vi "Add Constant or Error VI.vi"() -> ()   [LabVIEW 2020, in "ConstantErrorsMaker.lvlib"]
uses:
  Libraries/ConstantErrorsMaker/ConstantErrorsMaker.lvlib
  Libraries/ConstantErrorsMaker/VI to make Type--enum.ctl
panel:
  in  "Selection":T1
  in  "Cancel":bool
  in  "OK":bool
  in  "Target":u16(ring) items=["Project : To Test PDash.lvproj", "Library : My Singleton Module.lvlib", "Library : My Cloneable Module.lvlib", "Library : Application.lvlib", "Library : ConstantErrorsMaker.lvlib", "Class : SingletonClass.lvclass", "Class : CloneableClass.lvclass", "Class : Project Class.lvclass", "<Select a Module/Library/Project>"]
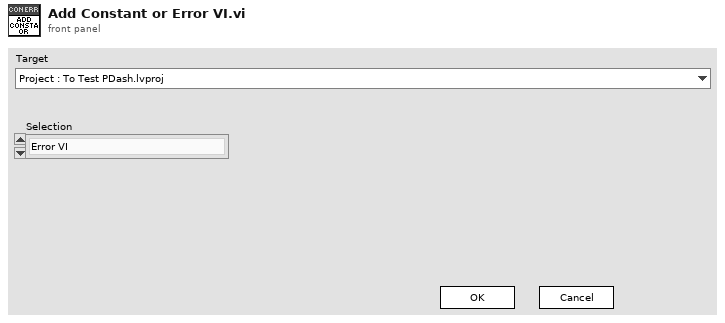
[diagram p1: front panel]
types:
  T1 = typedef "ConstantErrorsMaker.lvlib/VI to make Type--enum.ctl" = enum16{"Error VI", "Constant VI"}
  T2 = typedef "ConstantErrorsMaker.lvlib/Selection Info--cluster.ctl" = cluster{"Name":string, "Library Ref":refnum<vi>, "Application Instance":refnum<vi>, "Selection Owning Folder":path, "Selection Type":T3, "Project Reference":refnum<vi>, "LVClassLibrary Refnum":refnum<vi>}
  T3 = typedef "ConstantErrorsMaker.lvlib/Selection Type--enum.ctl" = enum16{"Project", "Library", "Class"}
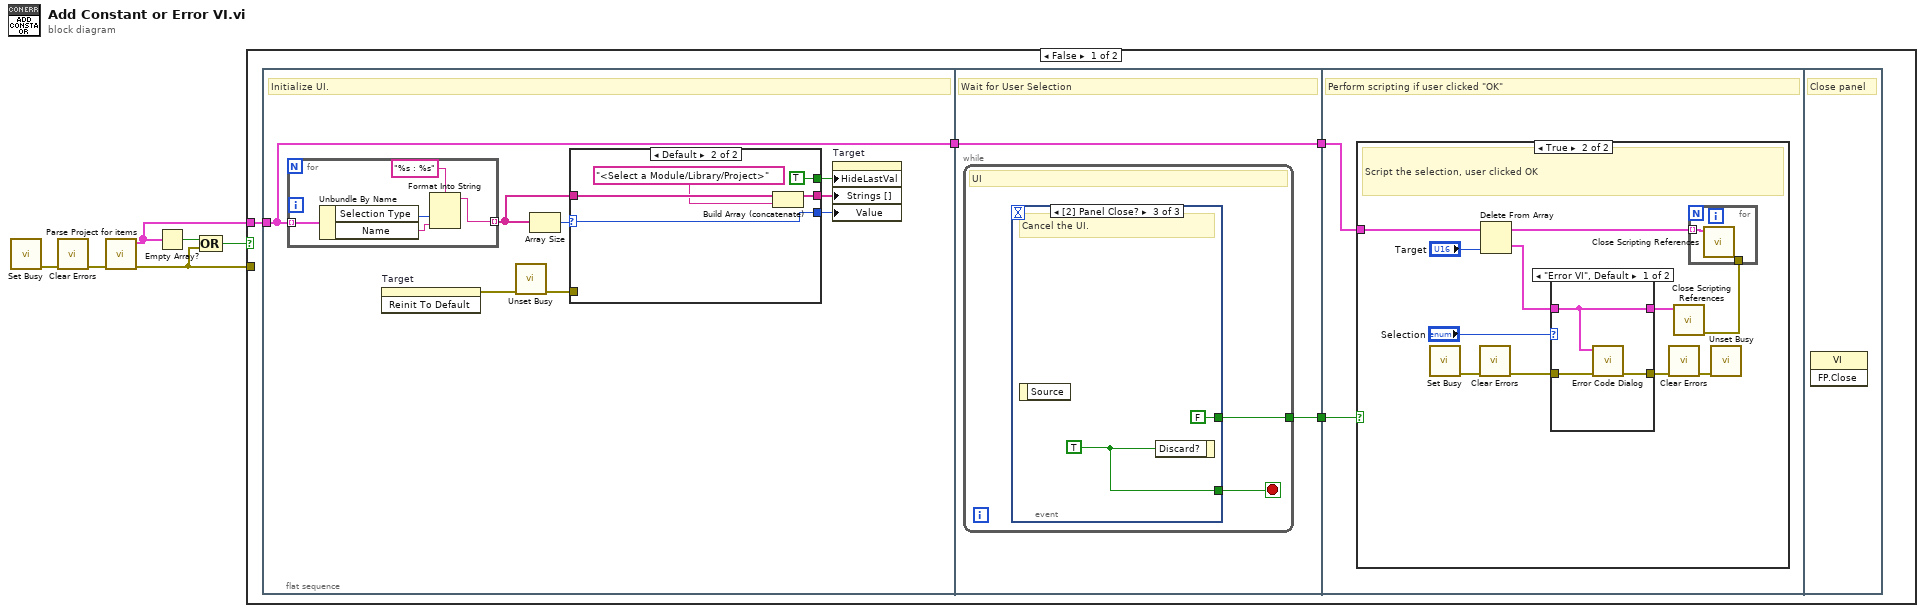
[diagram p0: block diagram]
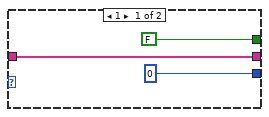
[diagram p2: hidden frame]
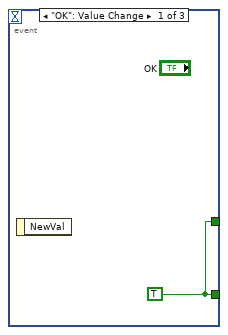
[diagram p3: hidden frame]
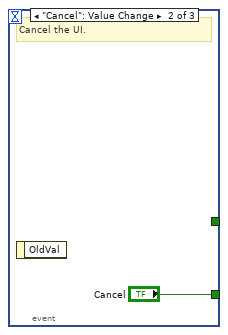
[diagram p4: hidden frame]
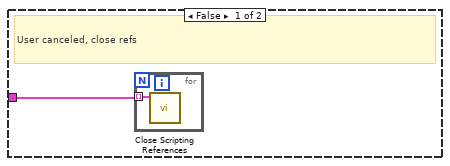
[diagram p5: hidden frame]
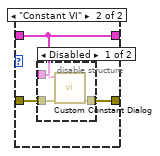
[diagram p6: hidden frame]
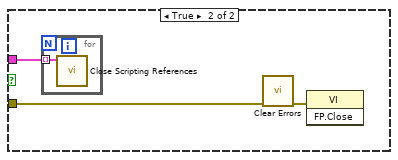
[diagram p8: hidden frame]
diagram:
  n1 = call <vilib>:"Set Busy.vi"() -> ("error out"=w5:errorcluster)  [unwired: 10 in, 1 out]
  n2 = call <vilib>:"Clear Errors.vi"("error in (no error)"=w5) -> ("error out"=w4:errorcluster)  [unwired: 5 in, 1 out]
  n3 = call "Parse Project for items.vi"("error in"=w4) -> ("error out"=w6:errorcluster, "Items"=w1:T2[])  [unwired: 9 in]
  n4 = Empty Array?(array=w1) -> (empty?=w3:bool)
  n5 = Compound Arithmetic op=OR(w3, w6) -> (w2:bool)
  n6 = case shown="False" w2 {
    tunnel: w6 -> [_ w67]
    tunnel: w1 -> [w10 w65]
    frame False {
      n7 = flat-sequence {
        tunnel: w10 -> [w11]
        tunnel: [w11] -> w9
        tunnel: w9 -> [w33]
        tunnel: [w33] -> w8
        tunnel: [w32] -> w7
        tunnel: w8 -> [w41]
        tunnel: w7 -> [w40]
        frame #0 {
          # "Initialize UI."
          n8 = for {
            tunnel: w11 -> [w31] mode=indexing
            tunnel: [w30] -> w15 mode=indexing
            n9 = Unbundle By Name(w31) -> ("Selection Type"=w28:T3, "Name"=w29:string)
            n10 = Format Into String(format string="%s : %s", w28, w29) -> (resulting string=w30:string)  [unwired: 2 in, 1 out]
          }
          n11 = invoke on="Target" class="Ring (strict)" method="Reinit To Default"() -> (error out=w17:errorcluster)  [unwired: 3 in, 2 out]
          n12 = call <vilib>:"Unset Busy.vi"("error in (no error)"=w17) -> ("error out"=w18:errorcluster)  [unwired: 10 in]
          n13 = Array Size(array=w15) -> (size(s)=w12:i32)
          n14 = case shown="Default" w12 {
            selector: w12 -> [_ w23]
            tunnel: [FALSE ("Hide Last Value") TRUE ("Hide Last Value")] -> w16
            tunnel: w15 -> [w21 w25]
            tunnel: [w21 w24] -> w14
            tunnel: [0 w23] -> w13
            tunnel: w18 -> [_ _]
            frame 1 {
            }
            frame Default {
              n15 = Build Array (concatenate)(w25, "<Select a Module/Library/Project>") -> (w24:string[])
            }
          }
          n16 = property on="Target" class="Ring (strict)"("HideLastVal"=w16, "Strings []"=w14, "Value"=w13) -> ()  [unwired: 2 in, 2 out]
        }
        frame #1 {
          # "Wait for User Selection"
          n17 = while {
            tunnel: [w35] -> w32
            stop <- w34 stop-if-true
            # "UI"
            n18 = event shown="[2] Panel Close?" {
              selector: _ -> [_ _ _]
              dyn-events: _ -> [_ _ _]
              timeout: _ -> [_ _ _]
              tunnel: [w36 "Cancel" w39] -> w34
              tunnel: [w36 _ FALSE ("OK to Proceed?")] -> w35
              event "OK": Value Change {
                w36 = TRUE ("Discard?")
                n19 = event-data() -> ()  [unwired: 1 in, 1 out]
              }
              event "Cancel": Value Change {
                # "Cancel the UI."
                n20 = event-data() -> ()  [unwired: 1 in, 1 out]
              }
              event Panel Close? {
                w39 = TRUE ("Discard?")
                # "Cancel the UI."
                n21 = event-data() -> ()  [unwired: 1 in, 1 out]
                n22 = event-data("Discard?"=w39) -> ()  [unwired: 1 in, 1 out]
              }
            }
          }
        }
        frame #2 {
          # "Perform scripting if user clicked \"OK\""
          n23 = case shown="True" w40 {
            tunnel: w41 -> [w42 w50]
            frame False {
              # "User canceled, close refs"
              n24 = for {
                tunnel: w42 -> [w43] mode=indexing
                n25 = call "Close Scripting References.vi"("Selection Info"=w43) -> ()  [unwired: 10 in, 1 out]
              }
            }
            frame True {
              # "Script the selection, user clicked OK"
              n26 = call <vilib>:"Set Busy.vi"() -> ("error out"=w53:errorcluster)  [unwired: 10 in, 1 out]
              n27 = call <vilib>:"Clear Errors.vi"("error in (no error)"=w53) -> ("error out"=w52:errorcluster)  [unwired: 5 in, 1 out]
              n28 = Delete From Array(array=w50, index="Target") -> (deleted portion=w46:T2, array with subset deleted=w49:T2[])  [unwired: 1 in]
              n29 = case shown="\"Error VI\", Default" "Selection" {
                tunnel: w46 -> [w55 w58]
                tunnel: [w55 w58] -> w45
                tunnel: w52 -> [w57 w60]
                tunnel: [w56 w59] -> w51
                frame "Error VI", Default {
                  n30 = call "Error Code Dialog.vi"("error in"=w57, "Selection"=w55) -> ("error out"=w56:errorcluster)  [unwired: 8 in, 1 out]
                }
                frame "Constant VI" {
                  n31 = disable-structure shown="Disabled" {
                    disable-tunnel: w60 -> [w63 _]
                    disable-tunnel: [w62 _] -> w59
                    disable-tunnel: w58 -> [w61 _]
                    frame Disabled {
                      n32 = call "Custom Constant Dialog.vi"("error in"=w63, "Selection"=w61) -> ("error out"=w62:errorcluster)  [unwired: 7 in, 2 out]
                    }
                    frame Enabled {
                    }
                  }
                }
              }
              n33 = call <vilib>:"Clear Errors.vi"("error in (no error)"=w51) -> ("error out"=w54:errorcluster)  [unwired: 5 in, 1 out]
              n34 = call "Close Scripting References.vi"("Selection Info"=w45) -> ("error out"=w44:errorcluster)  [unwired: 10 in]
              n35 = for {
                tunnel: w49 -> [w64] mode=indexing
                tunnel: w44 -> [_]
                n36 = call "Close Scripting References.vi"("Selection Info"=w64) -> ()  [unwired: 10 in, 1 out]
              }
              n37 = call <vilib>:"Unset Busy.vi"("error in (no error)"=w54) -> ()  [unwired: 10 in, 1 out]
            }
          }
        }
        frame #3 {
          # "Close panel"
          n38 = invoke class="VI" method="FP.Close"() -> ()  [unwired: 3 in, 3 out]
        }
      }
    }
    frame True {
      n39 = for {
        tunnel: w65 -> [w68] mode=indexing
        n40 = call "Close Scripting References.vi"("Selection Info"=w68) -> ()  [unwired: 10 in, 1 out]
      }
      n41 = call <vilib>:"Clear Errors.vi"("error in (no error)"=w67) -> ("error out"=w66:errorcluster)  [unwired: 5 in, 1 out]
      n42 = invoke class="VI" method="FP.Close"(error in=w66) -> ()  [unwired: 2 in, 3 out]
    }
  }
